vi "AB_RW_Cache_Project_Path.vi"(7 "action":T2, 8 "error in (no error)":errorcluster, 10 "ProjectPath in":path, 11 "buildObject":T1) -> (0 "error out":errorcluster, 2 "ProjectPath out":path, 3 "buildObject out":T1)   [LabVIEW 2020]
doc: "Reads and writes the data to the object property bag."
uses:
  <resource>/Framework/Providers/API/ItemRef.ctl
  <vilib>/AppBuilder/RW_Project/AB_RW_Project_PropBag_Action.ctl
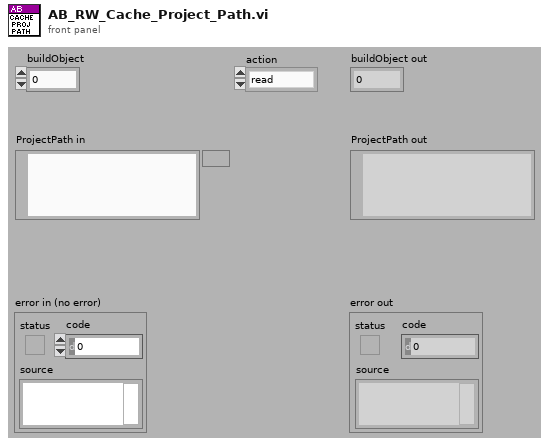
[diagram p1: front panel]
types:
  T1 = typedef "ItemRef.ctl" = u64
  T2 = typedef "AB_RW_Project_PropBag_Action.ctl" = enum16{"read", "write", "clear", "readPrevious", "writePrevious", "clearPrevious"}
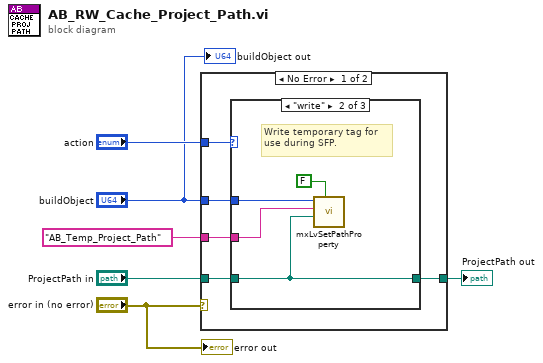
[diagram p0: block diagram]
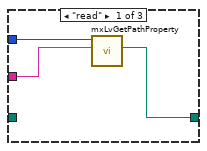
[diagram p2: hidden frame]
diagram:
  n1 = case shown="No Error" "error in (no error)" {
    tunnel: "action" -> [w11 _]
    tunnel: "buildObject" -> [w10 _]
    tunnel: "ProjectPath in" -> [w9 w20]
    tunnel: "AB_Temp_Project_Path" -> [w8 _]
    tunnel: [w7 w20] -> w1
    frame No Error {
      n2 = case shown="\"write\"" w11 {
        tunnel: w10 -> [w14 w18 _]
        tunnel: w9 -> [_ w15 w19]
        tunnel: w8 -> [w13 w17 _]
        tunnel: [w12 w15 w19] -> w7
        frame "read" {
          n3 = call <resource>:"mxLvGetPathProperty.vi"("Tag"=w13, "Item"=w14) -> ("Path"=w12:path)  [unwired: 2 in, 7 out]
        }
        frame "write" {
          # "Write temporary tag for use during SFP."
          n4 = call <resource>:"mxLvSetPathProperty.vi"("Persist Property? (T)"=FALSE, "Path"=w15, "Tag"=w17, "Item"=w18) -> ()  [unwired: 1 in, 7 out]
        }
        frame "clear", Default {
        }
      }
    }
    frame Error {
    }
  }
  "ProjectPath out" <- w1
  "error out" <- "error in (no error)"
  "buildObject out" <- "buildObject"
